vi "Control Label to PhXP Settings Element.vi"(1 "Label.Text":string) -> (0 "Settings List Element":T1)   [LabVIEW 2019]
uses:
  Phasor Explorer Settings List.ctl
panel:
  in  "PhXP Settings List":T1
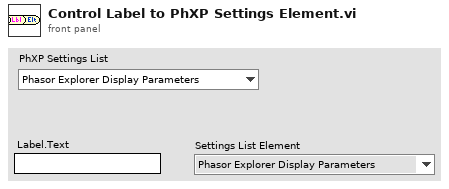
[diagram p1: front panel]
types:
  T1 = typedef "Phasor Explorer Settings List.ctl" = enum16{"Phasor Explorer Display Parameters", "Phasor Explorer Phasor Parameters", "Phasor Explorer Decay & IRF Parameters", "Phasor Explorer Gate Parameters", "Phasor Explorer Detector Parameters", "f*", "tau*"}
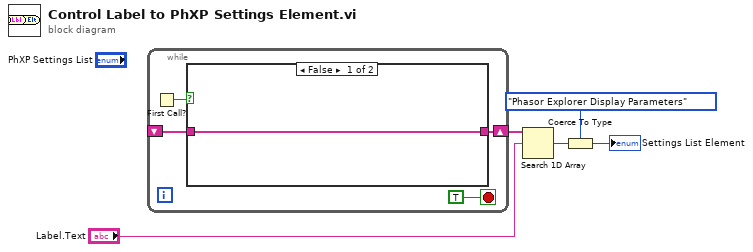
[diagram p0: block diagram]
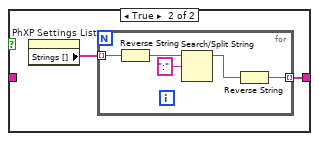
[diagram p2: hidden frame]
diagram:
  n1 = while {
    shift-right: [w7] -> w1
    shift-left: _ -> [w6]
    stop <- TRUE stop-if-true
    n2 = First Call?() -> (First Call?: T/F=w9:bool)
    n3 = case shown="False" w9 {
      tunnel: [w10 w12] -> w7
      tunnel: w6 -> [w10 _]
      frame False {
      }
      frame True {
        n4 = property on="PhXP Settings List" class="Enum (strict)"() -> ("Strings []"=w11:string[])  [unwired: 2 in, 2 out]
        n5 = for {
          tunnel: w11 -> [w17] mode=indexing
          tunnel: [w13] -> w12 mode=indexing
          n6 = Reverse String(1:w17) -> (0:w15:string)
          n7 = Search/Split String(string=w15, search string/char (-)=":") -> (substring before match=w14:string)  [unwired: 1 in, 2 out]
          n8 = Reverse String(1:w14) -> (0:w13:string)
        }
      }
    }
  }
  n9 = Search 1D Array(1D array=w1, element="Label.Text") -> (index of element=w3:i32)  [unwired: 1 in]
  n10 = Coerce To Type(0:w3, 1:Phasor_Explorer_Settings_List."Phasor Explorer Display Parameters" ("PhXP Settings List")) -> (2:→"Settings List Element":T1)
